vi "StepSizeSet.vi"(8 "error in (no error)":errorcluster, 10 "Desired Step Size":u8=1, 11 "VISA resource name":refnum<visa-resource-name>) -> (0 "error out":errorcluster, 2 "Command not accepted":bool, 3 "VISA resource name out":refnum<visa-resource-name>)   [LabVIEW 2017, in "Spectral Products CM110.lvlib"]
uses:
  Spectral Products CM110.lvlib
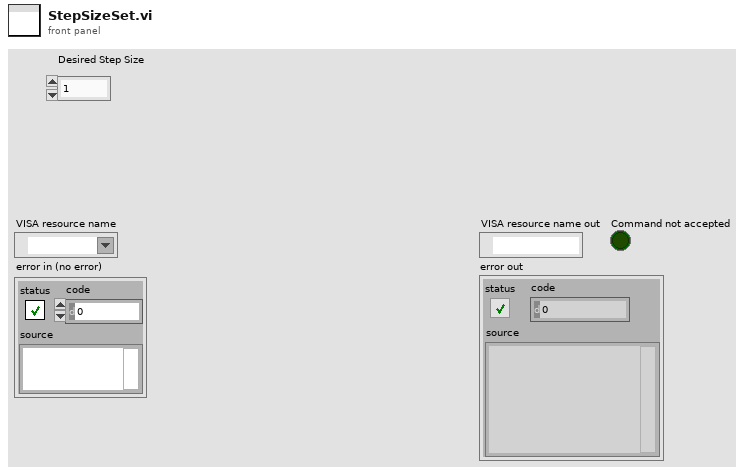
[diagram p1: front panel]
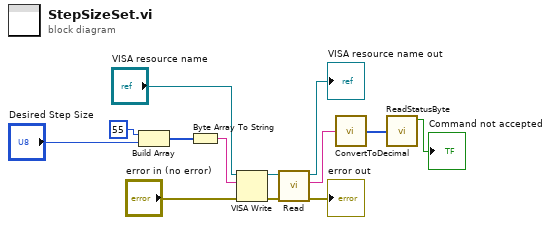
[diagram p0: block diagram]
diagram:
  n1 = Build Array(u8 55, "Desired Step Size") -> (w9:u8[])
  n2 = Byte Array To String(unsigned byte array=w9) -> (string=w8:string)
  n3 = VISA Write(VISA resource name="VISA resource name", write buffer=w8, error in (no error)="error in (no error)") -> (VISA resource name out=w6:refnum<visa-resource-name>, error out=w5:errorcluster)  [unwired: 1 out]
  n4 = call "Read.vi"("error in (no error)"=w5, "VISA Refnum in"=w6) -> ("error out"=→"error out":errorcluster, "read buffer"=w11:string, "VISA Refnum out"=→"VISA resource name out":refnum<visa-resource-name>)  [unwired: 6 in, 1 out]
  n5 = call "ConvertToDecimal.vi"("read buffer"=w11) -> ("unsigned byte array"=w7:u8[])
  n6 = call "ReadStatusByte.vi"("unsigned byte array"=w7) -> ("Command not accepted"=→"Command not accepted":bool)  [unwired: 4 in, 5 out]
